vi "AH2700Monitor.vi"() -> ()   [LabVIEW 2016]
uses:
  Instrument_Setup.vi
  Global/Global Variables/global.vi
  Global/Global Variables/Data_Display_global.vi
  Equipment/Capacity_Bridge_AH2700A/Andeen-Hagerling 2700/Andeen-Hagerling 2700.lvlib
panel:
  in  "Total":i32 min=0 max=99999999
  in  "Interval":dbl min=0.0 max=99999999.0 step=0.1 format="%#_10f"
  in  "stop":bool
  out "Capacitance":dbl format="%#_10f"
  out "Loss":dbl
  out "Applied Voltage":dbl format="%#_6f"
  out "Error Message":string
  out "Frequency":dbl
  out "Sample Switch":i32
  out "Units Display":i32(ring)=1 items=["nanosiemens"=1, "dissipation factor"=2, "kilohms"=3, "gigohms"=4, "loss vector (jpF)"=5]
  in  "Serial Configuration":T1={"Baud Rate"=9600, "Parity"=0, "Data Bits"=8, "Stop Bits"=10} {"Stop Bits" items=["1.0"=10, "1.5"=15, "2.0"=20]; "Data Bits" items=["7"=7, "8"=8]; "Parity" items=["None", "Odd", "Even", "Mark", "Space"]; "Baud Rate" items=["300"=300, "600"=600, "1200"=1200, "2400"=2400, "4800"=4800, "9600"=9600, "19200"=19200]}
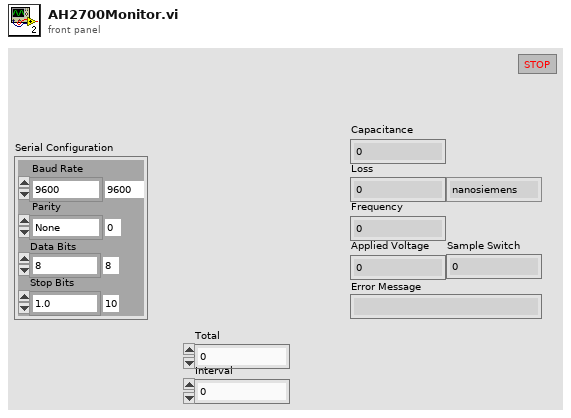
[diagram p1: front panel]
types:
  T1 = cluster{"Baud Rate":u32, "Parity":u16, "Data Bits":u16, "Stop Bits":u16}
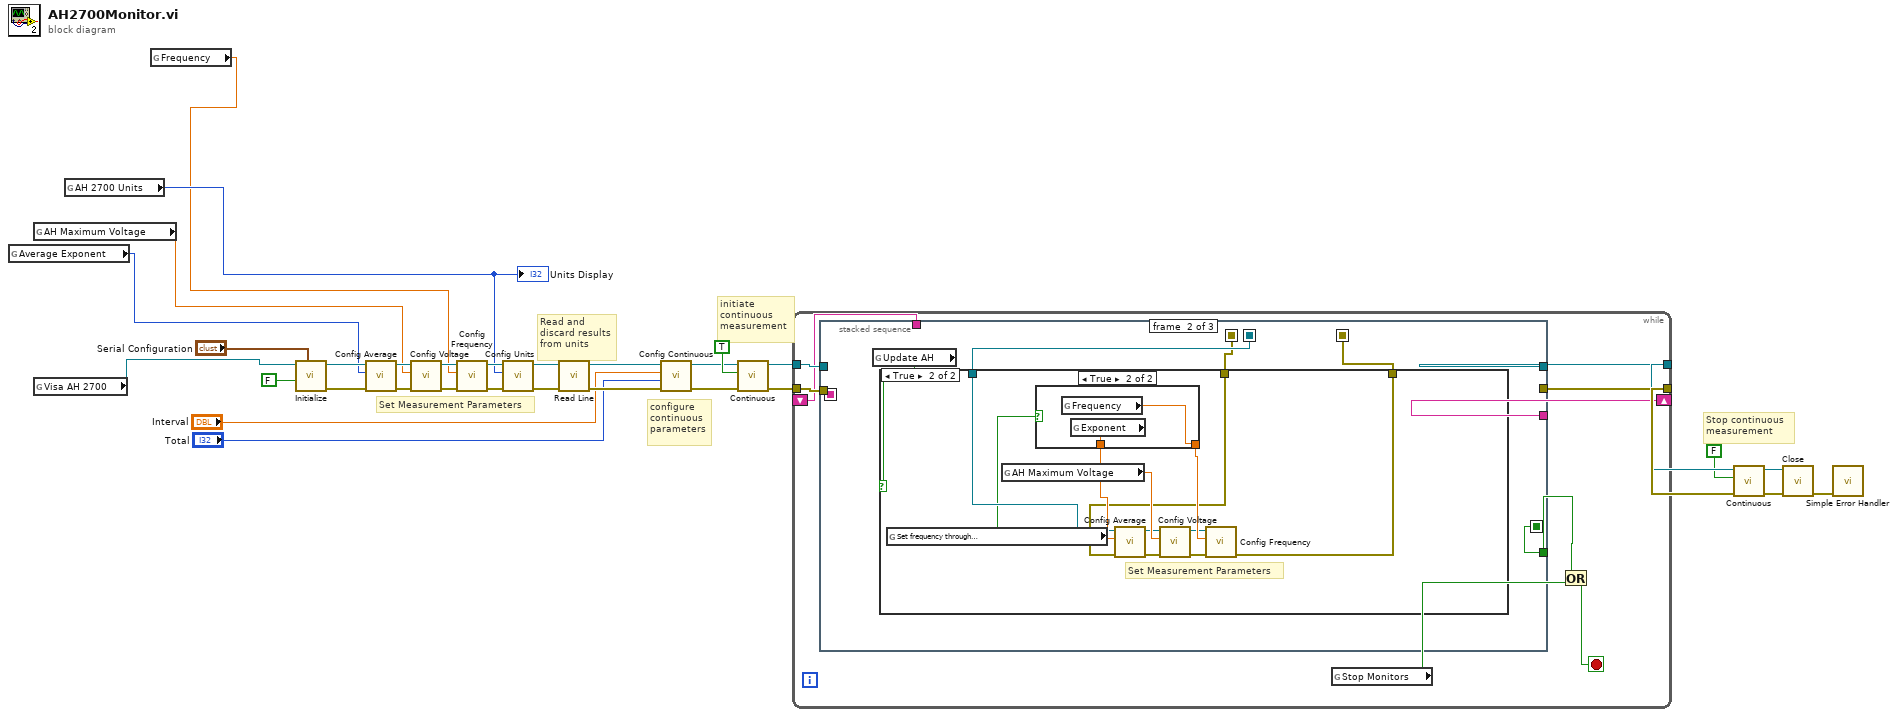
[diagram p0: block diagram]
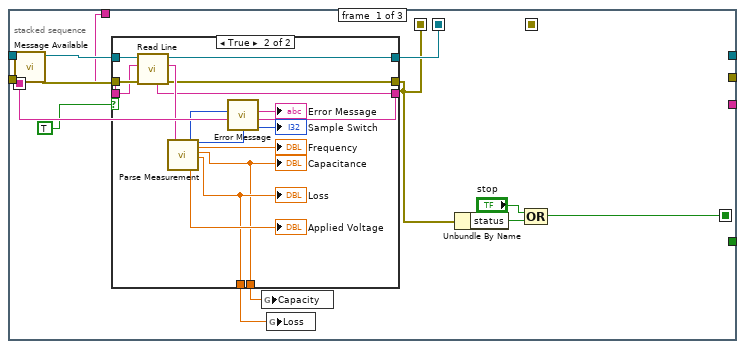
[diagram p2: hidden frame]
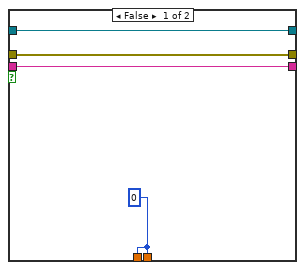
[diagram p3: hidden frame]
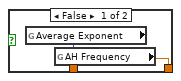
[diagram p5: hidden frame]
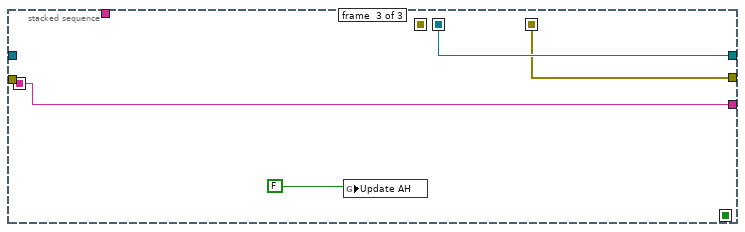
[diagram p6: hidden frame]
diagram:
  # "configure\ncontinuous\nparameters"
  # "Stop continuous\nmeasurement"
  # "initiate\ncontinuous\nmeasurement"
  # "Set Measurement Parameters"
  # "Read and\ndiscard results\nfrom units"
  n1 = global read "Instrument_Setup.vi" "Average Exponent"() -> (w3:u16)
  n2 = global read "Instrument_Setup.vi" "AH Maximum Voltage"() -> (w5:dbl)
  n3 = global read "Instrument_Setup.vi" "Visa AH 2700"() -> (w2:refnum<visa-resource-name>)
  n4 = global read "Instrument_Setup.vi" "AH 2700 Units"() -> (w4:i32)
  "Units Display" <- w4
  n5 = global read "global.vi" "Frequency"() -> (w1:dbl)
  n6 = call "Initialize.vi"("Serial Configuration"="Serial Configuration", "Reset (True)"=FALSE, "VISA resource name"=w2) -> ("error out"=w21:errorcluster, "VISA resource name out"=w22:refnum<visa-resource-name>)  [unwired: 7 in]
  n7 = call "Config Average.vi"("error in"=w21, "Average Exponent (4)"=w3, "VISA resource name"=w22) -> ("error out"=w27:errorcluster, "VISA resource name out"=w30:refnum<visa-resource-name>)  [unwired: 7 in]
  n8 = call "Config Voltage.vi"("error in"=w27, "Voltage (15 V)"=w5, "VISA resource name"=w30) -> ("error out"=w26:errorcluster, "VISA resource name out"=w29:refnum<visa-resource-name>)  [unwired: 7 in]
  n9 = call "Config Frequency.vi"("error in"=w26, "Frequency (1000 Hz)"=w1, "VISA resource name"=w29) -> ("error out"=w25:errorcluster, "VISA resource name out"=w28:refnum<visa-resource-name>)  [unwired: 7 in]
  n10 = call "Config Units.vi"("error in"=w25, "Units (nS)"=w4, "VISA resource name"=w28) -> ("error out"=w23:errorcluster, "VISA resource name out"=w24:refnum<visa-resource-name>)  [unwired: 7 in]
  n11 = call "Read Line.vi"("error in"=w23, "VISA resource name"=w24) -> ("error out"=w9:errorcluster, "VISA resource name out"=w11:refnum<visa-resource-name>)  [unwired: 5 in, 3 out]
  n12 = call "Config Continuous.vi"("error in"=w9, "Total (0)"="Total", "Interval (0)"="Interval", "VISA resource name"=w11) -> ("error out"=w8:errorcluster, "VISA resource name out"=w10:refnum<visa-resource-name>)  [unwired: 6 in]
  n13 = call "Continuous.vi"("error in"=w8, "Continuous Measurement (true)"=TRUE ("On (true)"), "VISA resource name"=w10) -> ("error out"=w19:errorcluster, "VISA resource name out"=w20:refnum<visa-resource-name>)  [unwired: 7 in]
  n14 = while {
    tunnel: [w41] -> w14
    tunnel: [w33] -> w16
    tunnel: w20 -> [w39]
    tunnel: w19 -> [w38]
    shift-right: [w40] -> _
    shift-left: _ -> [w37]
    stop <- w34 stop-if-true
    n15 = stacked-sequence {
      seq-local: [w55 _ _] -> [_ _ w97]
      seq-local: [w43 _ _] -> [_ w77 w96]
      seq-local: [w42 _ _] -> [_ w76 _]
      seq-local: [w49 _ _] -> [_ w74 _]
      seq-local: [_ w75 _] -> [_ _ w95]
      tunnel: w39 -> [w54 _ _]
      tunnel: w38 -> [w52 _ _]
      tunnel: w37 -> [w47 _ _]
      tunnel: [_ _ w96] -> w41
      tunnel: [_ _ w97] -> w40
      tunnel: [_ w74 _] -> w36
      tunnel: [_ _ w95] -> w33
      frame #0 {
        n16 = call "Message Available.vi"("error in"=w52, "VISA resource name"=w54) -> ("error out"=w51:errorcluster, "VISA resource name out"=w53:refnum<visa-resource-name>)  [unwired: 7 in, 1 out]
        n17 = case shown="True" TRUE {
          tunnel: [w59 w73] -> w43
          tunnel: w53 -> [w59 w70]
          tunnel: w51 -> [w58 w69]
          tunnel: [w58 w64] -> w42
          tunnel: [w57 w63] -> w55
          tunnel: w47 -> [w57 w62]
          tunnel: [w56 w61] -> w45
          tunnel: [w56 w60] -> w46
          frame False {
            w56 = 0
          }
          frame True {
            n18 = call "Read Line.vi"("error in"=w69, "Previous"=w62, "VISA resource name"=w70) -> ("error out"=w64:errorcluster, "Message"=w72:string, "VISA resource name out"=w73:refnum<visa-resource-name>, "Remaining"=w63:string)  [unwired: 4 in, 1 out]
            n19 = call "Parse Measurement.vi"("Measurement Line"=w72) -> ("Error Code"=w71:i32, "Voltage"=→"Applied Voltage":dbl, "Sample"=→"Sample Switch":i32, "Frequency"=→"Frequency":dbl, "Capacitance"=w60:dbl, "Loss"=w61:dbl)  [unwired: 10 in, 3 out]
            "Capacitance" <- w60
            "Loss" <- w61
            n20 = call "Error Message.vi"("Error Code"=w71) -> ("Error Message"=→"Error Message":string)  [unwired: 10 in]
          }
        }
        n21 = global write "Data_Display_global.vi" "Capacity"(w46) -> ()
        n22 = global write "Data_Display_global.vi" "Loss"(w45) -> ()
        n23 = Unbundle By Name(w42) -> ("status"=w50:bool)
        n24 = Compound Arithmetic op=OR("stop", w50) -> (w49:bool)
      }
      frame #1 {
        n25 = global read "Data_Display_global.vi" "Update AH"() -> (w78:bool)
        n26 = case shown="True" w78 {
          tunnel: w77 -> [_ w83]
          tunnel: w76 -> [w79 w82]
          tunnel: [w79 w81] -> w75
          frame False {
          }
          frame True {
            # "Set Measurement Parameters"
            n27 = global read "Instrument_Setup.vi" "Set frequency through\ncommand file"() -> (w80:bool)
            n28 = global read "Instrument_Setup.vi" "AH Maximum Voltage"() -> (w88:dbl)
            n29 = case shown="True" w80 {
              tunnel: [w91 w93] -> w90
              tunnel: [w92 w94] -> w89
              frame False {
                n30 = global read "Instrument_Setup.vi" "Average Exponent"() -> (w92:u16)
                n31 = global read "Instrument_Setup.vi" "AH Frequency"() -> (w91:dbl)
              }
              frame True {
                n32 = global read "global.vi" "Frequency"() -> (w93:dbl)
                n33 = global read "global.vi" "Exponent"() -> (w94:dbl)
              }
            }
            n34 = call "Config Average.vi"("error in"=w82, "Average Exponent (4)"=w89, "VISA resource name"=w83) -> ("error out"=w86:errorcluster, "VISA resource name out"=w84:refnum<visa-resource-name>)  [unwired: 7 in]
            n35 = call "Config Voltage.vi"("error in"=w86, "Voltage (15 V)"=w88, "VISA resource name"=w84) -> ("error out"=w87:errorcluster, "VISA resource name out"=w85:refnum<visa-resource-name>)  [unwired: 7 in]
            n36 = call "Config Frequency.vi"("error in"=w87, "Frequency (1000 Hz)"=w90, "VISA resource name"=w85) -> ("error out"=w81:errorcluster)  [unwired: 7 in, 1 out]
          }
        }
      }
      frame #2 {
        n37 = global write "Data_Display_global.vi" "Update AH"(FALSE) -> ()
      }
    }
    n38 = global read "Data_Display_global.vi" "Stop Monitors"() -> (w35:bool)
    n39 = Or(x=w36, y=w35) -> (x .or. y?=w34:bool)
  }
  n40 = call "Continuous.vi"("error in"=w16, "Continuous Measurement (true)"=FALSE ("On (true)"), "VISA resource name"=w14) -> ("error out"=w17:errorcluster, "VISA resource name out"=w15:refnum<visa-resource-name>)  [unwired: 7 in]
  n41 = call "Close.vi"("error in (no error)"=w17, "VISA resource name"=w15) -> ("error out"=w12:errorcluster)  [unwired: 9 in]
  n42 = call <vilib>:"Simple Error Handler.vi"("error in (no error)"=w12) -> ()  [unwired: 4 in, 5 out]
